vi "Post-Process.vi"(11 "Ship in":refnum<class "Ship.lvclass">) -> (3 "Ship out":refnum<class "Ship.lvclass">)   [LabVIEW 2021, in "Ship.lvclass"]
uses:
  Ship.lvclass
  Element/Element.lvclass
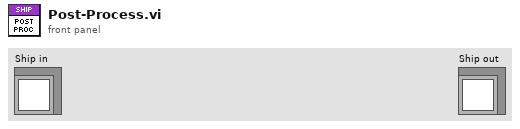
[diagram p1: front panel]
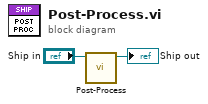
[diagram p0: block diagram]
diagram:
  n1 = call-parent "Post-Process.vi"("Element in"="Ship in") -> ("Element out"=→"Ship out":refnum<class "Ship.lvclass">)  [unwired: 10 in]
